vi "Writing_Reading.vi"(4 "Saving File Path":path, 5 "Enable":bool, 6 "Alarm_IN":bool, 8 "Length_IN":dbl, 9 "Speed_IN":dbl) -> (0 "Alarm_OUT":bool, 1 "data":string[][](array[string]), 2 "Length_OUT":dbl, 3 "Speed_OUT":dbl)   [LabVIEW 2020]
uses:
  <vilib>/Utility/NIReport.llb/Report Type.ctl
  <vilib>/express/express shared/transition.llb/Dynamic To Waveform Array.vi
  <vilib>/express/express signal manip/GetorSetDDTAttributes/Set DDT Attributes/SetT0.vi
  <vilib>/express/express shared/transition.llb/Waveform Array To Dynamic.vi
  <vilib>/addons/_office/excel.llb/Excel Get Data ([str]).vi
  <vilib>/express/express signal manip/GetorSetDDTAttributes/Set DDT Attributes/Set DDT Properties.xnode
  <vilib>/Utility/NIReport.llb/NI_report.lvclass
  <vilib>/Utility/NIReport.llb/NI_ReportGenerationCore.lvlib
  <vilib>/Utility/NIReport.llb/Excel/NI_Excel.lvclass
  <vilib>/addons/_office/NI_ReportGenerationToolkit.lvlib
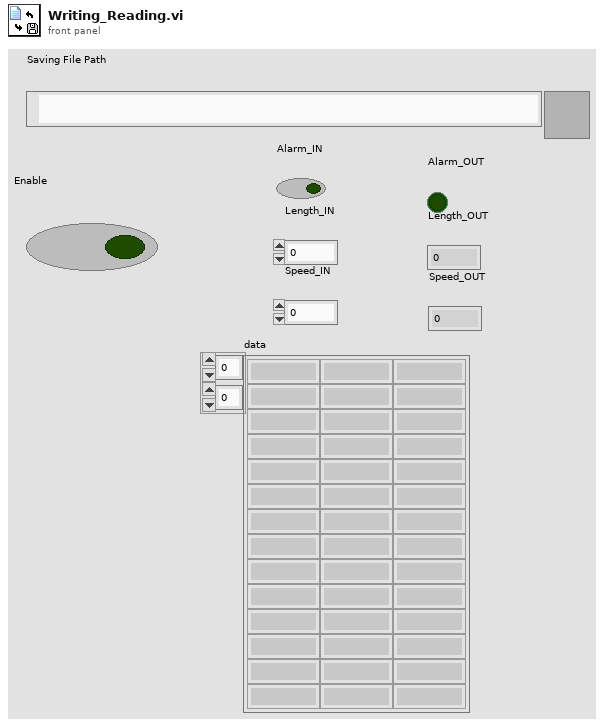
[diagram p1: front panel]
types:
  T1 = typedef "NI_ReportGenerationCore.lvlib/Report Type.ctl" = enum16{"HTML", "Word", "Excel"}
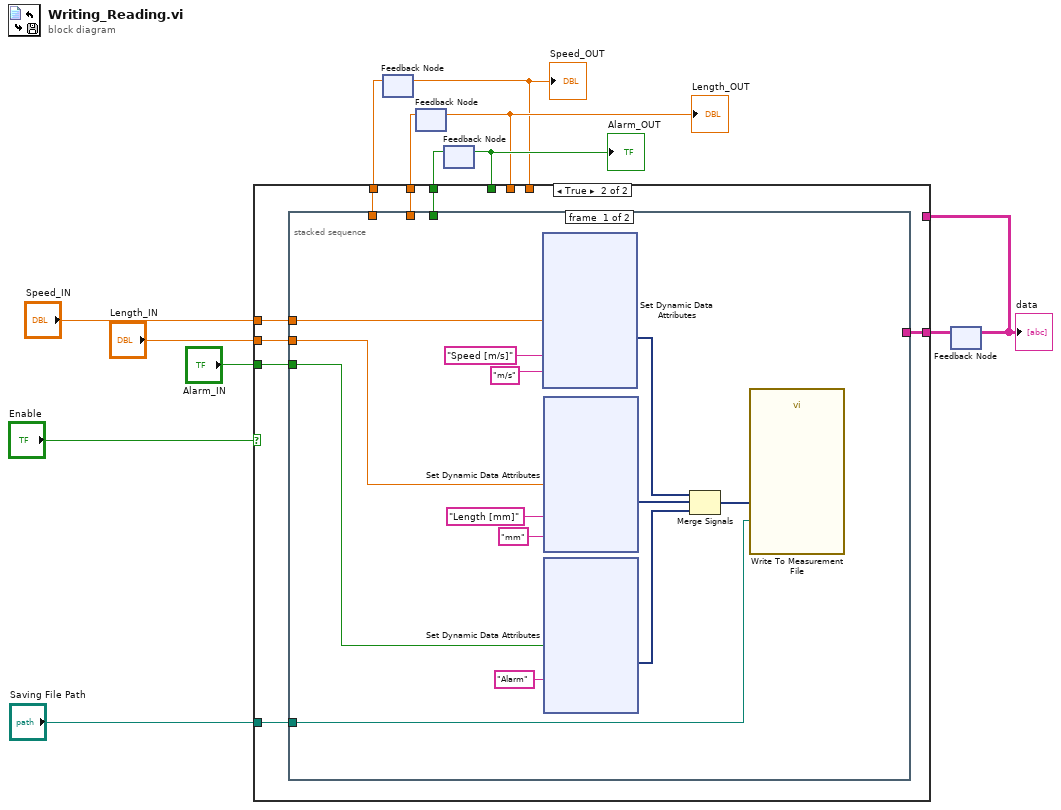
[diagram p0: block diagram]
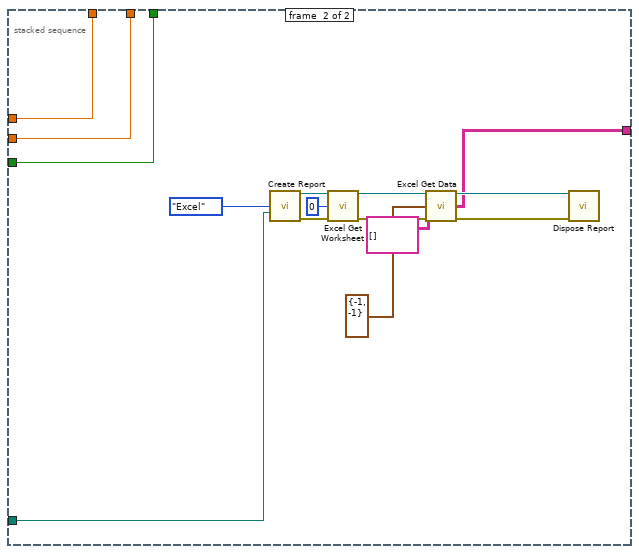
[diagram p3: hidden frame]
diagram:
  n1 = feedback #1() -> (w1:dbl)  [unwired: 1 in]
  "Speed_OUT" <- w1
  n2 = feedback #2() -> (w2:dbl)  [unwired: 1 in]
  "Length_OUT" <- w2
  n3 = feedback #3() -> (w3:bool)  [unwired: 1 in]
  "Alarm_OUT" <- w3
  n4 = feedback #4() -> (w10:string[][])  [unwired: 1 in]
  "data" <- w10
  n5 = case shown="True" "Enable" {
    tunnel: "Saving File Path" -> [_ w25]
    tunnel: [w17 w24] -> w11
    tunnel: w10 -> [w17 _]
    tunnel: "Alarm_IN" -> [_ w23]
    tunnel: "Length_IN" -> [_ w22]
    tunnel: "Speed_IN" -> [_ w21]
    tunnel: [w16 w20] -> w6
    tunnel: [w15 w19] -> w5
    tunnel: [w14 w18] -> w4
    tunnel: w3 -> [w14 _]
    tunnel: w2 -> [w15 _]
    tunnel: w1 -> [w16 _]
    frame False {
    }
    frame True {
      n6 = stacked-sequence {
        tunnel: w25 -> [w29 w97]
        tunnel: [_ w96] -> w24
        tunnel: w23 -> [w28 w95]
        tunnel: w22 -> [w27 w94]
        tunnel: w21 -> [w26 w93]
        tunnel: [_ w93] -> w20
        tunnel: [_ w94] -> w19
        tunnel: [_ w95] -> w18
        frame #0 {
          n7 = xnode "Set Dynamic Data Attributes"("Signals In"=w26, "Signal Name"="Speed [m/s]", "Unit"="m/s") -> ("Signals Out"=w34:dynamicdata)  [unwired: 2 in, 1 out]
          n8 = xnode "Set Dynamic Data Attributes"("Signals In"=w27, "Signal Name"="Length [mm]", "Unit"="mm") -> ("Signals Out"=w33:dynamicdata)  [unwired: 2 in, 1 out]
          n9 = xnode "Set Dynamic Data Attributes"("Signals In"=w28, "Signal Name"="Alarm") -> ("Signals Out"=w32:dynamicdata)  [unwired: 3 in, 1 out]
          n10 = Merge Signals(w34, w33, w32) -> (w31:dynamicdata)
          n11 = call "Write To Measurement File"("Signals"=w31, "Filename"=w29) -> ()  [unwired: 15 in, 3 out]
        }
        frame #1 {
          n12 = call <vilib>:"Create Report.vi"("report type"=Report_Type."Excel", "template (empty)"=w97) -> ("report out"=w105:refnum<class "NI_report.lvclass">, "error out"=w106:errorcluster)  [unwired: 12 in]
          n13 = call <vilib>:"Excel Get Worksheet.vi"("report in"=w105, "worksheet index (0)"=0, "error in (no error)"=w106) -> ("report out"=w103:refnum<class "NI_report.lvclass">, "error out"=w102:errorcluster)  [unwired: 11 in]
          n14 = call-poly <vilib>:"Excel Get Data.vi"("report in"=w103, "data type"=string[][] [], "start (-1, -1)"=cluster{"start row":i32, "start column":i32} {"start row"=-1, "start column"=-1} ("start (0, 0)"), "error in (no error)"=w102) -> ("report out"=w99:refnum<class "NI_report.lvclass">, "data"=w96:string[][], "error out"=w98:errorcluster)  [unwired: 9 in]
          n15 = call-dynamic "Dispose Report.vi"("report in"=w99, "error in (no error)"=w98) -> ()  [unwired: 13 in, 1 out]
        }
      }
    }
  }
  n16 = feedback-in #1(w6) -> ()
  n17 = feedback-in #2(w5) -> ()
  n18 = feedback-in #3(w4) -> ()
  n19 = feedback-in #4(w11) -> ()
